vi "LinearFilter_FiniteDifference.vi"(8 "Period":dbl=0.02, 9 "Stencil":i32[](array[numeric]), 11 "Derivative":i32) -> (0 "Error":bool, 3 "LINEAR_FILTER":T1 {"Outputs" format="%13.5g"; "Inputs" format="%13.5g"; "OutputGains" format="%13.5g"; "InputGains" format="%13.5g"})   [LabVIEW 2019, in "Trajectory_Library.lvlib"]
doc: "Creates a finite difference filter that computes the nth derivative of the input given the specified stencil points.\n \nStencil points are the indices of the samples to use in the finite difference. 0 is the current sample, -1 is the previous sample, -2 is the sample before that, etc. Don't use positive stencil points (samples from the future) if the LinearFilter will be used for stream-based online filtering.\n\nFor additional information see:\n https://en.wikipedia.org/wiki/Finite_difference_coefficient#Arbitrary_stencil_points\n \nFor a given list of stencil points s of length n and the order of derivative d < n, the finite difference coefficients can be obtained by solving the following linear system for the vector a.\n\n [s1° ? s?° ][a1] [ d0,d ]\n [ ? ? ? ][? ] = d! [ ? ]\n [s1n?¹ ? s?n?¹][a?] [d??1,d]\n \n where d?,? are the Kronecker delta. The FIR gains are the elements of the\n vector a in reverse order divided by h?.\n \n The order of accuracy of the approximation is of the form O(hn??).\n\nInputs: \n - derivative -- The order of the derivative to compute.\n - stencil -- Lisst of stencil points. Its length is the number of samples to use to compute the given derivative. This must be one more than the order of the derivative or higher.\n - period -- The period in seconds between samples taken by the user.\n\nOutputs:\n - LINEAR FILTER - cluster containing:\n - InputGains - Array of “feedforward” or FIR gain factors (bx)\n - OutputGains - Array of “feedback” or IIR gain factors for feedback terms (ax)\n - Inputs - Array of the last n saved inputs\n - Outputs - Array of the last n saved outputs\n - InGainCount - Number of input gain terms\n - OutGainCount - number of output gain terms\n - Error -- Returns TRUE if an error occured."
uses:
  Trajectory_Library.lvlib
  <vilib>/Analysis/NI_AALPro.lvlib
  <vilib>/Analysis/7linalg.llb/Solve Linear Equations (multiple right hand).vi
  TypeDef/LINEAR_FILTER.ctl
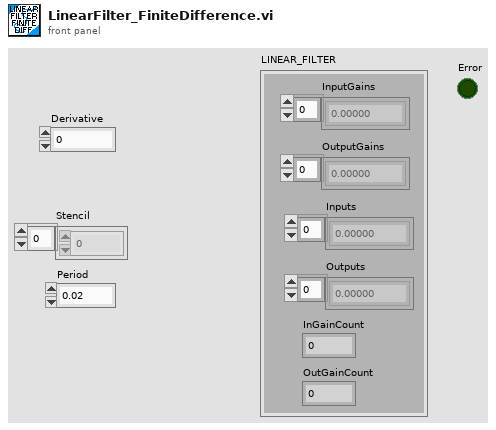
[diagram p1: front panel]
types:
  T1 = typedef "Trajectory_Library.lvlib/LINEAR_FILTER.ctl" = cluster{"InputGains":dbl[], "OutputGains":dbl[], "Inputs":dbl[], "Outputs":dbl[], "InGainCount":i32, "OutGainCount":i32}
  T2 = typedef "NI_Matrix.lvlib/RealMatrix.ctl" = dbl[][]
  T3 = typedef "WPILib_Math.lvlib/LINEAR_FILTER.ctl" = cluster{"InputGains":dbl[], "OutputGains":dbl[], "Inputs":dbl[], "Outputs":dbl[], "InGainCount":i32, "OutGainCount":i32}
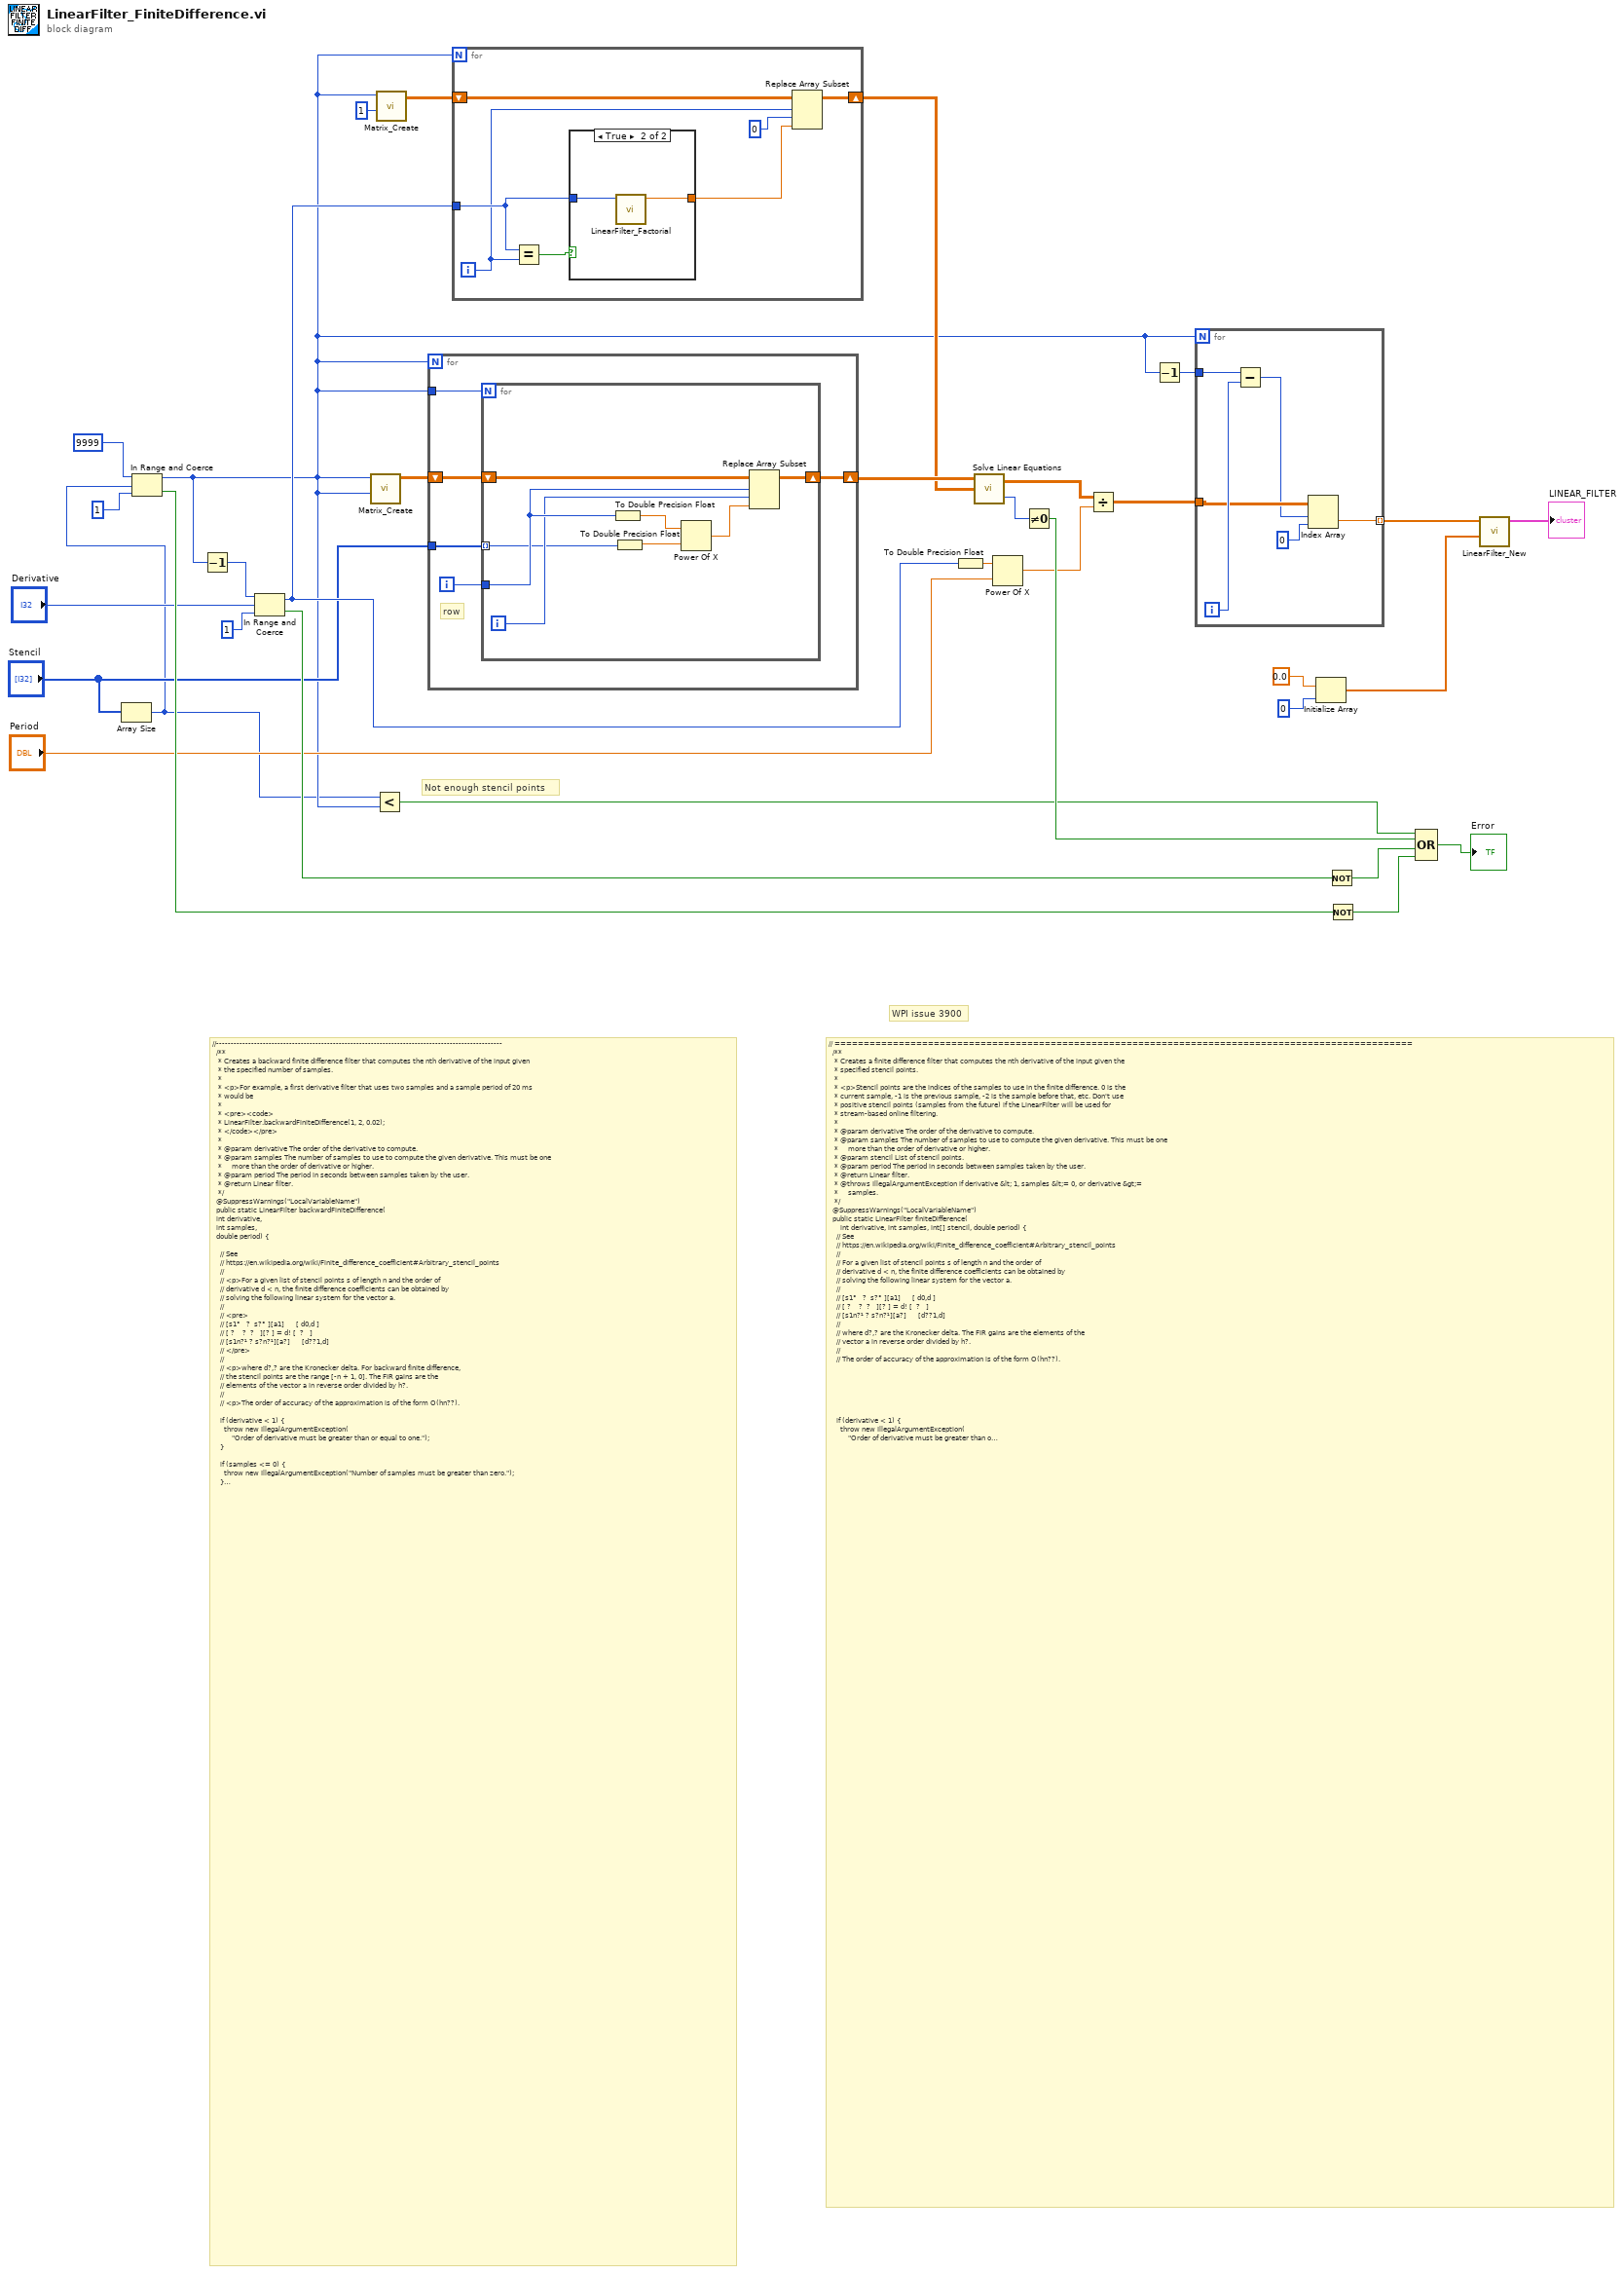
[diagram p0: block diagram]
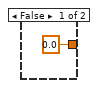
[diagram p2: hidden frame]
diagram:
  # "Not enough stencil points"
  # "WPI issue 3900"
  # "// ===================================================================================================\n  /**\n   * Creates a finite difference filter that computes the nth derivative of the input given the\n   * specified stencil points.\n   *\n   * <p>Stencil points are the indices of the samples to use in the finite difference. 0 is the\n   * current sample, -1 is the previous sample, -2 is the sample before that, etc. Don't use\n   * positive stencil points (samples from the future) if the LinearFilter will be used for\n   * stream-based online filtering.\n   *\n   * @param derivative The order of the derivative to compute.\n   * @param samples The number of samples to use to compute the given derivative. This must be one\n   *     more than the order of derivative or higher.\n   * @param stencil List of stencil points.\n   * @param period The period in seconds between samples taken by the user.\n   * @return Linear filter.\n   * @throws IllegalArgumentException if derivative &lt; 1, samples &lt;= 0, or derivative &gt;=\n   *     samples.\n   */\n  @SuppressWarnings(\"LocalVariableName\")\n  public static LinearFilter finiteDifference(\n      int derivative, int samples, int[] stencil, double period) {\n    // See\n    // https://en.wikipedia.org/wiki/Finite_difference_coefficient#Arbitrary_stencil_points\n    //\n    // For a given list of stencil points s of length n and the order of\n    // derivative d < n, the finite difference coefficients can be obtained by\n    // solving the following linear system for the vector a.\n    //\n    // [s1°   ?  s?° ][a1]      [ d0,d ]\n    // [ ?    ?  ?   ][? ] = d! [  ?   ]\n    // [s1n?¹ ? s?n?¹][a?]      [d??1,d]\n    //\n    // where d?,? are the Kronecker delta. The FIR gains are the elements of the\n    // vector a in reverse order divided by h?.\n    //\n    // The order of accuracy of the approximation is of the form O(hn??).\n\n\n\n\n\n\n    if (derivative < 1) {\n      throw new IllegalArgumentException(\n          \"Order of derivative must be greater than or equal to one.\");\n    }\n\n    if (samples <= 0) {\n      throw new IllegalArgumentException(\"Number of samples must be greater than zero.\");\n    }\n\n    if (derivative >= samples) {\n      throw new IllegalArgumentException(\n          \"Order of derivative must be less than number of samples.\");\n    }\n\n    var S = new SimpleMatrix(samples, samples);\n    for (int row = 0; row < samples; ++row) {\n      for (int col = 0; col < samples; ++col) {\n        S.set(row, col, Math.pow(stencil[col], row));\n      }\n    }\n\n    // Fill in Kronecker deltas: https://en.wikipedia.org/wiki/Kronecker_delta\n    var d = new SimpleMatrix(samples, 1);\n    for (int i = 0; i < samples; ++i) {\n      d.set(i, 0, (i == derivative) ? factorial(derivative) : 0.0);\n    }\n\n    var a = S.solve(d).divide(Math.pow(period, derivative));\n\n    // Reverse gains list\n    double[] ffGains = new double[samples];\n    for (int i = 0; i < samples; ++i) {\n      ffGains[i] = a.get(samples - i - 1, 0);\n    }\n\n    return new LinearFilter(ffGains, new double[0]);\n  }"
  # "//--------------------------------------------------------------------------------------------------\n  /**\n   * Creates a backward finite difference filter that computes the nth derivative of the input given\n   * the specified number of samples.\n   *\n   * <p>For example, a first derivative filter that uses two samples and a sample period of 20 ms\n   * would be\n   *\n   * <pre><code>\n   * LinearFilter.backwardFiniteDifference(1, 2, 0.02);\n   * </code></pre>\n   *\n   * @param derivative The order of the derivative to compute.\n   * @param samples The number of samples to use to compute the given derivative. This must be one\n   *     more than the order of derivative or higher.\n   * @param period The period in seconds between samples taken by the user.\n   * @return Linear filter.\n   */\n  @SuppressWarnings(\"LocalVariableName\")\n  public static LinearFilter backwardFiniteDifference(\n\t\tint derivative, \n\t\tint samples, \n\t\tdouble period) {\n\n    // See\n    // https://en.wikipedia.org/wiki/Finite_difference_coefficient#Arbitrary_stencil_points\n    //\n    // <p>For a given list of stencil points s of length n and the order of\n    // derivative d < n, the finite difference coefficients can be obtained by\n    // solving the following linear system for the vector a.\n    //\n    // <pre>\n    // [s1°   ?  s?° ][a1]      [ d0,d ]\n    // [ ?    ?  ?   ][? ] = d! [  ?   ]\n    // [s1n?¹ ? s?n?¹][a?]      [d??1,d]\n    // </pre>\n    //\n    // <p>where d?,? are the Kronecker delta. For backward finite difference,\n    // the stencil points are the range [-n + 1, 0]. The FIR gains are the\n    // elements of the vector a in reverse order divided by h?.\n    //\n    // <p>The order of accuracy of the approximation is of the form O(hn??).\n\n    if (derivative < 1) {\n      throw new IllegalArgumentException(\n          \"Order of derivative must be greater than or equal to one.\");\n    }\n\n    if (samples <= 0) {\n      throw new IllegalArgumentException(\"Number of samples must be greater than zero.\");\n    }\n\n    if (derivative >= samples) {\n      throw new IllegalArgumentException(\n          \"Order of derivative must be less than number of samples.\");\n    }\n\n    var S = new SimpleMatrix(samples, samples);\n    for (int row = 0; row < samples; ++row) {\n      for (int col = 0; col < samples; ++col) {\n        double s = 1 - samples + col;\n        S.set(row, col, Math.pow(s, row));\n      }\n    }\n\n    // Fill in Kronecker deltas: https://en.wikipedia.org/wiki/Kronecker_delta\n    var d = new SimpleMatrix(samples, 1);\n    for (int i = 0; i < samples; ++i) {\n      d.set(i, 0, (i == derivative) ? factorial(derivative) : 0.0);\n    }\n\n    var a = S.solve(d).divide(Math.pow(period, derivative));\n\n    // Reverse gains list\n    double[] ffGains = new double[samples];\n    for (int i = 0; i < samples; ++i) {\n      ffGains[i] = a.get(samples - i - 1, 0);\n    }\n\n    double[] fbGains = new double[0];\n\n    return new LinearFilter(ffGains, fbGains);\n  }"
  n1 = Array Size(array="Stencil") -> (size(s)=w1:i32)
  n2 = In Range and Coerce(upper limit=9999, x=w1, lower limit=1) -> (coerced(x)=w3:i32, In Range?=w31:bool)
  n3 = Decrement(x=w3) -> (x-1=w29:i32)
  n4 = In Range and Coerce(upper limit=w29, x="Derivative", lower limit=1) -> (coerced(x)=w12:i32, In Range?=w27:bool)
  n5 = call "Matrix_Create.vi"("Columns"=w3, "Rows"=w3) -> ("output matrix"=w23:T2)  [unwired: 9 in]
  n6 = Less?(x=w1, y=w3) -> (x < y?=w2:bool)
  n7 = call "Matrix_Create.vi"("Columns"=1, "Rows"=w3) -> ("output matrix"=w21:T2)  [unwired: 9 in]
  n8 = for {
    N: w3 -> [_]
    shift-right: [w35] -> w20
    shift-left: w23 -> [w37]
    tunnel: w3 -> [w38]
    tunnel: "Stencil" -> [w34]
    i -> [w36]
    # "row"
    n9 = for {
      N: w38 -> [_]
      shift-right: [w45] -> w35
      shift-left: w37 -> [w46]
      tunnel: w36 -> [w44]
      tunnel: w34 -> [w40] mode=indexing
      i -> [w41]
      n10 = To Double Precision Float(number=w44) -> (double precision float=w43:dbl)
      n11 = To Double Precision Float(number=w40) -> (double precision float=w39:dbl)
      n12 = Power Of X(1:w39, 2:w43) -> (0:w42:dbl)
      n13 = Replace Array Subset(array=w46, new element=w42, index (row)=w44, index (col)=w41) -> (w45:T2)
    }
  }
  n14 = for {
    N: w3 -> [_]
    shift-right: [w52] -> w19
    shift-left: w21 -> [w53]
    tunnel: w12 -> [w50]
    i -> [w49]
    n15 = Equal?(x=w50, y=w49) -> (x = y?=w51:bool)
    n16 = case shown="True" w51 {
      tunnel: w50 -> [_ w56]
      tunnel: [0.0 ("Factorial") w55] -> w47
      frame False {
      }
      frame True {
        n17 = call "LinearFilter_Factorial.vi"("N"=w56) -> ("Factorial"=w55:dbl)  [unwired: 10 in]
      }
    }
    n18 = Replace Array Subset(array=w53, new element=w47, index (row)=w49, index (col)=0 ("disabled index (col)")) -> (w52:T2)
  }
  n19 = To Double Precision Float(number=w12) -> (double precision float=w17:dbl)
  n20 = call-poly <vilib>:"Solve Linear Equations.vi"("Known Matrix"=w19, "Input Matrix"=w20) -> ("error"=w16:i32, "Solution Matrix"=w14:T2)  [unwired: 1 in]
  n21 = Power Of X(1:"Period", 2:w17) -> (0:w13:dbl)
  n22 = Not Equal To 0?(x=w16) -> (x != 0?=w15:bool)
  n23 = Divide(x=w14, y=w13) -> (x/y=w11:T2)
  n24 = Decrement(x=w3) -> (x-1=w10:i32)
  n25 = for {
    N: w3 -> [_]
    tunnel: w11 -> [w60]
    tunnel: w10 -> [w62]
    tunnel: [w57] -> w7 mode=indexing
    i -> [w61]
    n26 = Subtract(x=w62, y=w61) -> (x-y=w59:i32)
    n27 = Index Array(array=w60, index (row)=w59, index (col)=0) -> (element=w57:dbl)
  }
  n28 = Initialize Array(0.0 ("element"), 0 ("dimension size")) -> (w6:dbl[])
  n29 = Not(x=w27) -> (.not. x?=w25:bool)
  n30 = Not(x=w31) -> (.not. x?=w26:bool)
  n31 = Compound Arithmetic op=OR(w2, w15, w25, w26) -> (→"Error":bool)
  n32 = call "LinearFilter_New.vi"("OutputGains"=w6, "InputGains"=w7) -> ("LINEAR_FILTER"=→"LINEAR_FILTER":T3)  [unwired: 9 in]
